vi "runSingle.vi"(8 "error in (no error)":errorcluster, 11 "HWController in":refnum<class "HWController.lvclass">) -> (0 "error out":errorcluster, 1 "devicesConfigured":string[](array[string]), 2 "Stopped":bool, 3 "HWController out":refnum<class "HWController.lvclass">)   [LabVIEW 2009, in "Hardware.lvlib" / "HWControllers.lvlib" / "HWController.lvclass"]
uses:
  HWController.lvclass
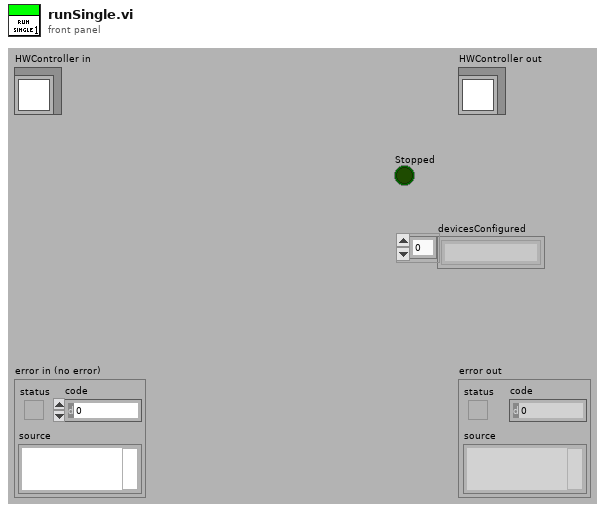
[diagram p1: front panel]
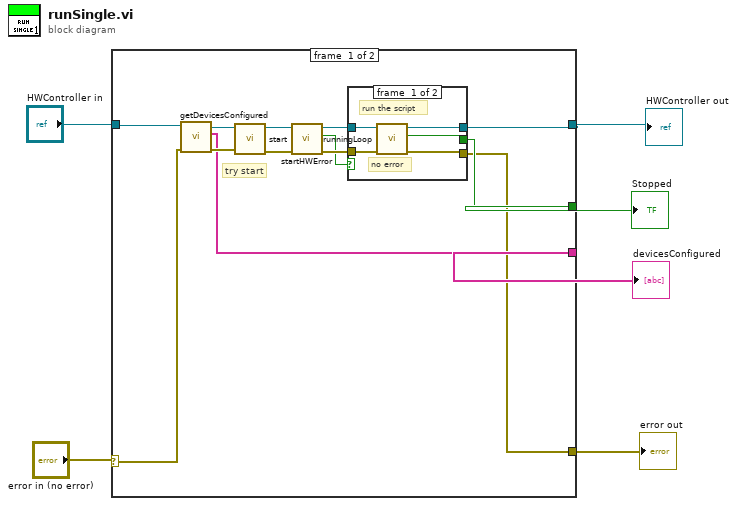
[diagram p0: block diagram]
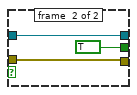
[diagram p2: hidden frame]
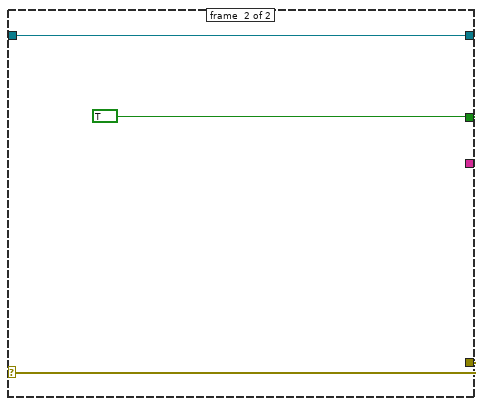
[diagram p3: hidden frame]
diagram:
  n1 = case shown="No Error" "error in (no error)" {
    selector: "error in (no error)" -> [w15 w30]
    tunnel: [w17 w30] -> w5
    tunnel: [w18 w29] -> w3
    tunnel: "HWController in" -> [w16 w29]
    tunnel: [w19 TRUE] -> w2
    tunnel: [w12 _] -> w1
    frame #0 {
      # "try start"
      n2 = call "getDevicesConfigured.vi"("error in (no error)"=w15, "HWController.lvclass in"=w16) -> ("error out"=w14:errorcluster, "devicesConfigured"=w12:string[], "HWController.lvclass out"=w13:refnum<class "HWController.lvclass">)  [unwired: 7 in]
      n3 = call-dynamic "start.vi"("error in (no error)"=w14, "HWController in"=w13) -> ("error out"=w11:errorcluster, "HWController out"=w10:refnum<class "HWController.lvclass">)  [unwired: 7 in, 1 out]
      n4 = call-dynamic "startHWError.vi"("error in (no error)"=w11, "HWController in"=w10) -> ("error out"=w8:errorcluster, "error"=w7:bool, "HWController out"=w9:refnum<class "HWController.lvclass">)  [unwired: 7 in]
      n5 = case shown="False" w7 {
        tunnel: [w24 TRUE] -> w19
        tunnel: [w23 w27] -> w18
        tunnel: [w22 w26] -> w17
        tunnel: w9 -> [w21 w27]
        tunnel: w8 -> [w20 w26]
        frame #0 {
          # "no error"
          # "run the script"
          n6 = call "runningLoop.vi"("error in (no error)"=w20, "HWController in"=w21) -> ("error out"=w22:errorcluster, "userStoped"=w24:bool, "HWController out"=w23:refnum<class "HWController.lvclass">)  [unwired: 7 in]
        }
        frame #1 {
        }
      }
    }
    frame #1 {
    }
  }
  "error out" <- w5
  "HWController out" <- w3
  "Stopped" <- w2
  "devicesConfigured" <- w1
